vi "test_firebase_db2.vi"() -> ()   [LabVIEW 2016]
uses:
  <vilib>/httpClient/PUTBuffer.vi
  <vilib>/httpClient/LabVIEWHTTPClient.lvlib
panel:
  in  "test":cluster{"name":string, "val":dbl, "onoff":bool}={"name"="ybbaek", "val"=42.0, "onoff"=TRUE}
  in  "data_table":T1={"test"={"name"="ybbaek", "val"=42.0, "onoff"=TRUE}, "motor"={"onoff"=FALSE, "pos"=3.163265306122449}} {"motor"."pos" scale=0.0..10.0}
  out "test_db":cluster{"name":string, "val":dbl, "onoff":bool}={"name"="ybbaek", "val"=42.0, "onoff"=TRUE}
  in  "R/W":bool=TRUE
  out "json_string":string="{\"test\":{\"name\":\"ybbaek\",\"val\":42,\"onoff\":true},\"motor\":{\"onoff\":false,\"pos\":3.1632653061224492}}"
  out "body":string="{\"motor\":{\"onoff\":false,\"pos\":3.163265306122449},\"test\":{\"name\":\"ybbaek\",\"onoff\":true,\"val\":42}}"
  out "headers":string="HTTP/1.1 100 Continue\r\n\r\nHTTP/1.1 200 OK\r\nServer: nginx\r\nDate: Wed, 25 Apr 2018 07:14:49 GMT\r\nContent-Type: application/json; charset=utf-8\r\nContent-Length: 96\r\nConnection: keep-alive\r\nAccess-Control-Allow-Origin: *\r\nCache-Control: no-cache\r\nStrict-Transport-Security: max-age=31556926; includeSubDomains; preload\r\n\r\n" caption="header"
  out "error out":errorcluster caption="에러 출력"
  in  "정지":bool
  in  "Firebase url":string="https://motlab-81406.firebaseio.com/.json"
  # "LabVIEW - Firebase DB"
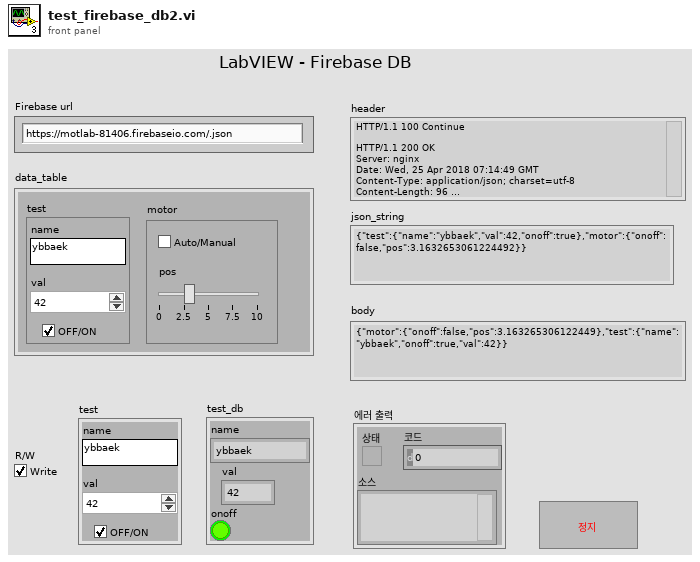
[diagram p1: front panel]
types:
  T1 = cluster{"test":cluster{"name":string, "val":dbl, "onoff":bool}, "motor":cluster{"onoff":bool, "pos":dbl}}
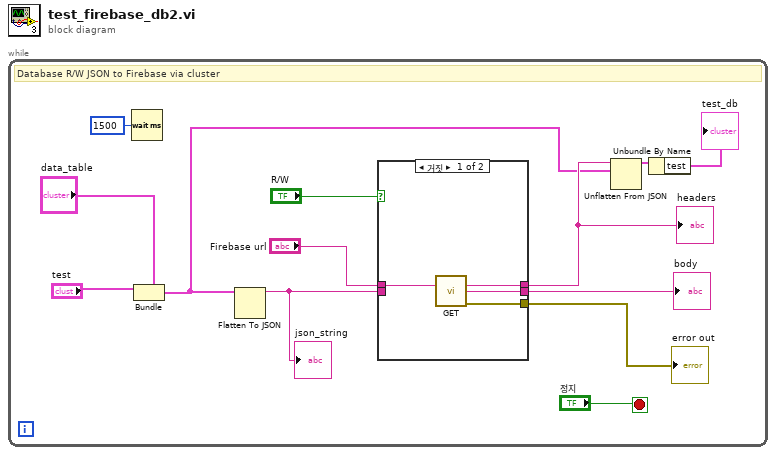
[diagram p0: block diagram]
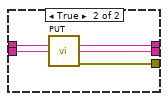
[diagram p2: hidden frame]
diagram:
  n1 = while {
    stop <- "정지" stop-if-true
    # "Database R/W JSON to Firebase via cluster"
    n2 = Wait (ms)(milliseconds to wait=u32 1500) -> ()  [unwired: 1 out]
    n3 = Bundle(cluster="data_table", "test"="test") -> (w3:T1)  [unwired: 1 in]
    n4 = Flatten To JSON(anything=w3) -> (JSON string=w8:string)  [unwired: 2 in, 1 out]
    "json_string" <- w8
    n5 = case shown="거짓" "R/W" {
      tunnel: "Firebase url" -> [w17 w22]
      tunnel: [w16 w21] -> w10
      tunnel: [w14 w20] -> w6
      tunnel: [w15 w19] -> w9
      tunnel: w8 -> [_ w18]
      frame False {
        n6 = call <vilib>:"GET.vi"("url"=w17) -> ("headers"=w14:string, "body"=w15:string, "error out"=w16:errorcluster)  [unwired: 11 in, 1 out]
      }
      frame True {
        n7 = call-poly <vilib>:"PUT.vi"("url"=w22, "buffer"=w18) -> ("headers"=w20:string, "body"=w19:string, "error out"=w21:errorcluster)  [unwired: 10 in, 1 out]
      }
    }
    "error out" <- w10
    "headers" <- w6
    "body" <- w9
    n8 = Unflatten From JSON(JSON string=w6, type and defaults=w3) -> (value=w2:T1)  [unwired: 5 in, 1 out]
    n9 = Unbundle By Name(w2) -> ("test"=→"test_db":cluster{"name":string, "val":dbl, "onoff":bool})
  }
